vi "WILT Agilent Populate GUI.vi"(7 "Aisle Number":T6=enum."Aisle 1", 8 "Error In":errorcluster, 10 "GUI Aisle Input":T3[](array[typedef]) {"Night Cycle Count" format="%04d"; "Day Cycle Count" format="%04d"}, 11 "Data Array":T1) -> (0 "Error Out":errorcluster, 3 "GUI Aisle Output":T3[](array[typedef]) {"Night Cycle Count" format="%04d"; "Day Cycle Count" format="%04d"}, 5 "Agilent Failure":bool)   [LabVIEW 2016]
uses:
  Type Definitions/WILT Aisle Number.ctl
  Type Definitions/WILT Agilent Channel Definition.ctl
  Type Definitions/WILT DAQ Data.ctl
  Type Definitions/WILT Dryer.ctl
  Type Definitions/WILT Dryer Details.ctl
  Type Definitions/WILT Agilent Data Cluster.ctl
panel:
  out "Index of stations that use\nthe same voltage":string[][](array[string])
  in  "Tab Control":enum32{"Check Information"}(tab)
  out "DAQ Data":T5={"L1 Current"=1.0, "L2 Current"=11.0, "Temperature  Deg F (TC)"=0.0, "Volts"=0.0, "Volts (208)"=0.0, "SW (208)"=0.0}
  out "DAQ Data 2":T5={"L1 Current"=2.0, "L2 Current"=22.0, "Temperature  Deg F (TC)"=0.0, "Volts"=0.0, "Volts (208)"=0.0, "SW (208)"=0.0}
  out "DAQ Data 3":T5={"L1 Current"=3.0, "L2 Current"=33.0, "Temperature  Deg F (TC)"=0.0, "Volts"=0.0, "Volts (208)"=0.0, "SW (208)"=0.0}
  out "DAQ Data 4":T5={"L1 Current"=4.0, "L2 Current"=44.0, "Temperature  Deg F (TC)"=0.0, "Volts"=0.0, "Volts (208)"=0.0, "SW (208)"=0.0}
  out "DAQ Data 5":T5={"L1 Current"=5.0, "L2 Current"=55.0, "Temperature  Deg F (TC)"=0.0, "Volts"=0.0, "Volts (208)"=0.0, "SW (208)"=0.0}
  out "DAQ Data 6":T5={"L1 Current"=6.0, "L2 Current"=66.0, "Temperature  Deg F (TC)"=0.0, "Volts"=0.0, "Volts (208)"=0.0, "SW (208)"=0.0}
  out "DAQ Data 7":T5
  out "DAQ Data 8":T5
  out "DAQ Data 9":T5
  out "DAQ Data 10":T5
  out "DAQ Data 11":T5
  out "DAQ Data 12":T5
  in  "Data Array (Old)":T2[](array[typedef])=[{"Channel"="101", "Station"="1", "Label"="L1 Current", "Agilent Station"="1", "Data"=1.0}, {"Channel"="102", "Station"="1", "Label"="L2 Current", "Agilent Station"="1", "Data"=11.0}, {"Channel"="103", "Station"="2", "Label"="L1 Current", "Agilent Station"="1", "Data"=2.0}, {"Channel"="104", "Station"="2", "Label"="L2 Current", "Agilent Station"="1", "Data"=22.0}, {"Channel"="105", "Station"="3", "Label"="L1 Current", "Agilent Station"="1", "Data"=3.0}, {"Channel"="106", "Station"="3", "Label"="L2 Current", "Agilent Station"="1", "Data"=33.0}, {"Channel"="107", "Station"="4", "Label"="L1 Current", "Agilent Station"="1", "Data"=4.0}, {"Channel"="108", "Station"="4", "Label"="L2 Current", "Agilent Station"="1", "Data"=44.0}, {"Channel"="109", "Station"="5", "Label"="L1 Current", "Agilent Station"="1", "Data"=5.0}, {"Channel"="110", "Station"="5", "Label"="L2 Current", "Agilent Station"="1", "Data"=55.0}, {"Channel"="111", "Station"="6", "Label"="L1 Current", "Agilent Station"="1", "Data"=6.0}, {"Channel"="112", "Station"="6", "Label"="L2 Current", "Agilent Station"="1", "Data"=66.0}, {"Channel"="113", "Station"="7", "Label"="L1 Current", "Agilent Station"="1", "Data"=7.0}, {"Channel"="114", "Station"="7", "Label"="L2 Current", "Agilent Station"="1", "Data"=77.0}, {"Channel"="115", "Station"="8", "Label"="L1 Current", "Agilent Station"="1", "Data"=8.0}, {"Channel"="116", "Station"="8", "Label"="L2 Current", "Agilent Station"="1", "Data"=88.0}, {"Channel"="201", "Station"="9", "Label"="L1 Current", "Agilent Station"="1", "Data"=9.0}, {"Channel"="202", "Station"="9", "Label"="L2 Current", "Agilent Station"="1", "Data"=99.0}, {"Channel"="203", "Station"="10", "Label"="L1 Current", "Agilent Station"="1", "Data"=10.0}, {"Channel"="204", "Station"="10", "Label"="L2 Current", "Agilent Station"="1", "Data"=1010.0}, {"Channel"="205", "Station"="11", "Label"="L1 Current", "Agilent Station"="1", "Data"=11.0}, {"Channel"="206", "Station"="11", "Label"="L2 Current", "Agilent Station"="1", "Data"=1111.0}, {"Channel"="207", "Station"="12", "Label"="L1 Current", "Agilent Station"="1", "Data"=12.0}, {"Channel"="208", "Station"="12", "Label"="L2 Current", "Agilent Station"="1", "Data"=1212.0}, {"Channel"="209", "Station"="13", "Label"="L1 Current", "Agilent Station"="1", "Data"=13.0}, {"Channel"="210", "Station"="13", "Label"="L2 Current", "Agilent Station"="1", "Data"=1313.0}, {"Channel"="211", "Station"="14", "Label"="L1 Current", "Agilent Station"="1", "Data"=14.0}, {"Channel"="212", "Station"="14", "Label"="L2 Current", "Agilent Station"="1", "Data"=1414.0}, {"Channel"="213", "Station"="15", "Label"="L1 Current", "Agilent Station"="1", "Data"=15.0}, {"Channel"="214", "Station"="15", "Label"="L2 Current", "Agilent Station"="1", "Data"=1515.0}, {"Channel"="215", "Station"="16", "Label"="L1 Current", "Agilent Station"="1", "Data"=16.0}, {"Channel"="216", "Station"="16", "Label"="L2 Current", "Agilent Station"="1", "Data"=1616.0}, {"Channel"="301", "Station"="17", "Label"="L1 Current", "Agilent Station"="1", "Data"=17.0}, {"Channel"="302", "Station"="17", "Label"="L2 Current", "Agilent Station"="1", "Data"=1717.0}, {"Channel"="303", "Station"="18", "Label"="L1 Current", "Agilent Station"="1", "Data"=18.0}, {"Channel"="304", "Station"="18", "Label"="L2 Current", "Agilent Station"="1", "Data"=1818.0}, {"Channel"="305", "Station"="19", "Label"="L1 Current", "Agilent Station"="1", "Data"=19.0}, {"Channel"="306", "Station"="19", "Label"="L2 Current", "Agilent Station"="1", "Data"=1919.0}, {"Channel"="307", "Station"="20", "Label"="L1 Current", "Agilent Station"="1", "Data"=0.0}, {"Channel"="308", "Station"="20", "Label"="L2 Current", "Agilent Station"="1", "Data"=0.0}, {"Channel"="309", "Station"="21", "Label"="L1 Current", "Agilent Station"="1", "Data"=0.0}, {"Channel"="310", "Station"="21", "Label"="L2 Current", "Agilent Station"="1", "Data"=0.0}, {"Channel"="311", "Station"="22", "Label"="L1 Current", "Agilent Station"="1", "Data"=0.0}, {"Channel"="312", "Station"="22", "Label"="L2 Current", "Agilent Station"="1", "Data"=0.0}, {"Channel"="313", "Station"="23", "Label"="L1 Current", "Agilent Station"="1", "Data"=0.0}, {"Channel"="314", "Station"="23", "Label"="L2 Current", "Agilent Station"="1", "Data"=0.0}, {"Channel"="315", "Station"="24", "Label"="L1 Current", "Agilent Station"="1", "Data"=0.0}, {"Channel"="316", "Station"="24", "Label"="L2 Current", "Agilent Station"="1", "Data"=0.0}, {"Channel"="101", "Station"="25", "Label"="L1 Current", "Agilent Station"="2", "Data"=0.0}, {"Channel"="102", "Station"="25", "Label"="L2 Current", "Agilent Station"="2", "Data"=0.0}, {"Channel"="103", "Station"="26", "Label"="L1 Current", "Agilent Station"="2", "Data"=0.0}, {"Channel"="104", "Station"="26", "Label"="L2 Current", "Agilent Station"="2", "Data"=0.0}, {"Channel"="105", "Station"="27", "Label"="L1 Current", "Agilent Station"="2", "Data"=0.0}, {"Channel"="106", "Station"="27", "Label"="L2 Current", "Agilent Station"="2", "Data"=0.0}, {"Channel"="107", "Station"="28", "Label"="L1 Current", "Agilent Station"="2", "Data"=0.0}, {"Channel"="108", "Station"="28", "Label"="L2 Current", "Agilent Station"="2", "Data"=0.0}, {"Channel"="109", "Station"="29", "Label"="L1 Current", "Agilent Station"="2", "Data"=0.0}, {"Channel"="110", "Station"="29", "Label"="L2 Current", "Agilent Station"="2", "Data"=0.0}, {"Channel"="111", "Station"="30", "Label"="L1 Current", "Agilent Station"="2", "Data"=0.0}, {"Channel"="112", "Station"="30", "Label"="L2 Current", "Agilent Station"="2", "Data"=0.0}, {"Channel"="113", "Station"="31", "Label"="L1 Current", "Agilent Station"="2", "Data"=0.0}, {"Channel"="114", "Station"="31", "Label"="L2 Current", "Agilent Station"="2", "Data"=0.0}, {"Channel"="115", "Station"="32", "Label"="L1 Current", "Agilent Station"="2", "Data"=0.0}, {"Channel"="116", "Station"="32", "Label"="L2 Current", "Agilent Station"="2", "Data"=0.0}, {"Channel"="201", "Station"="5", "Label"="Volts", "Agilent Station"="2", "Data"=555.0}, {"Channel"="202", "Station"="6", "Label"="Volts", "Agilent Station"="2", "Data"=666.0}, {"Channel"="203", "Station"="7", "Label"="Volts", "Agilent Station"="2", "Data"=777.0}, {"Channel"="204", "Station"="8", "Label"="Volts", "Agilent Station"="2", "Data"=888.0}, {"Channel"="205", "Station"="9", "Label"="Volts", "Agilent Station"="2", "Data"=999.0}, {"Channel"="206", "Station"="10", "Label"="Volts", "Agilent Station"="2", "Data"=101010.0}, {"Channel"="207", "Station"="11", "Label"="Volts", "Agilent Station"="2", "Data"=111111.0}, {"Channel"="208", "Station"="12", "Label"="Volts", "Agilent Station"="2", "Data"=121212.0}, {"Channel"="209", "Station"="13", "Label"="Volts", "Agilent Station"="2", "Data"=0.0}, {"Channel"="210", "Station"="14", "Label"="Volts", "Agilent Station"="2", "Data"=0.0}, {"Channel"="211", "Station"="21-23", "Label"="Volts", "Agilent Station"="2", "Data"=0.0}, {"Channel"="212", "Station"="24-26", "Label"="Volts", "Agilent Station"="2", "Data"=0.0}, {"Channel"="213", "Station"="27-29", "Label"="Volts", "Agilent Station"="2", "Data"=0.0}, {"Channel"="214", "Station"="30-32", "Label"="Volts", "Agilent Station"="2", "Data"=0.0}, {"Channel"="215", "Station"="15", "Label"="Volts", "Agilent Station"="2", "Data"=0.0}, {"Channel"="216", "Station"="16", "Label"="Volts", "Agilent Station"="2", "Data"=0.0}, {"Channel"="201", "Station"="1", "Label"="Temperature", "Agilent Station"="3", "Data"=1.0}, {"Channel"="202", "Station"="2", "Label"="Temperature", "Agilent Station"="3", "Data"=2.0}, {"Channel"="203", "Station"="3", "Label"="Temperature", "Agilent Station"="3", "Data"=3.0}, {"Channel"="204", "Station"="4", "Label"="Temperature", "Agilent Station"="3", "Data"=4.0}, {"Channel"="205", "Station"="5", "Label"="Temperature", "Agilent Station"="3", "Data"=5.0}, {"Channel"="206", "Station"="6", "Label"="Temperature", "Agilent Station"="3", "Data"=6.0}, {"Channel"="207", "Station"="7", "Label"="Temperature", "Agilent Station"="3", "Data"=7.0}, {"Channel"="208", "Station"="8", "Label"="Temperature", "Agilent Station"="3", "Data"=8.0}, {"Channel"="209", "Station"="9", "Label"="Temperature", "Agilent Station"="3", "Data"=9.0}, {"Channel"="210", "Station"="10", "Label"="Temperature", "Agilent Station"="3", "Data"=10.0}, {"Channel"="211", "Station"="11", "Label"="Temperature", "Agilent Station"="3", "Data"=11.0}, {"Channel"="212", "Station"="12", "Label"="Temperature", "Agilent Station"="3", "Data"=12.0}, {"Channel"="213", "Station"="13", "Label"="Temperature", "Agilent Station"="3", "Data"=0.0}, {"Channel"="214", "Station"="14", "Label"="Temperature", "Agilent Station"="3", "Data"=0.0}, {"Channel"="215", "Station"="15", "Label"="Temperature", "Agilent Station"="3", "Data"=0.0}, {"Channel"="216", "Station"="16", "Label"="Temperature", "Agilent Station"="3", "Data"=0.0}, {"Channel"="217", "Station"="17", "Label"="Temperature", "Agilent Station"="3", "Data"=0.0}, {"Channel"="218", "Station"="18", "Label"="Temperature", "Agilent Station"="3", "Data"=0.0}, {"Channel"="219", "Station"="19", "Label"="Temperature", "Agilent Station"="3", "Data"=0.0}, {"Channel"="220", "Station"="20", "Label"="Temperature", "Agilent Station"="3", "Data"=0.0}, {"Channel"="301", "Station"="21", "Label"="Temperature", "Agilent Station"="3", "Data"=0.0}, {"Channel"="302", "Station"="22", "Label"="Temperature", "Agilent Station"="3", "Data"=0.0}, {"Channel"="303", "Station"="23", "Label"="Temperature", "Agilent Station"="3", "Data"=0.0}, {"Channel"="304", "Station"="24", "Label"="Temperature", "Agilent Station"="3", "Data"=0.0}, {"Channel"="305", "Station"="25", "Label"="Temperature", "Agilent Station"="3", "Data"=0.0}, {"Channel"="306", "Station"="26", "Label"="Temperature", "Agilent Station"="3", "Data"=0.0}, {"Channel"="307", "Station"="27", "Label"="Temperature", "Agilent Station"="3", "Data"=0.0}, {"Channel"="308", "Station"="28", "Label"="Temperature", "Agilent Station"="3", "Data"=0.0}, {"Channel"="309", "Station"="29", "Label"="Temperature", "Agilent Station"="3", "Data"=0.0}, {"Channel"="310", "Station"="30", "Label"="Temperature", "Agilent Station"="3", "Data"=0.0}, {"Channel"="311", "Station"="31", "Label"="Temperature", "Agilent Station"="3", "Data"=0.0}, {"Channel"="312", "Station"="32", "Label"="Temperature", "Agilent Station"="3", "Data"=0.0}, {"Channel"="313", "Station"="1", "Label"="Volts", "Agilent Station"="3", "Data"=111.0}, {"Channel"="314", "Station"="2", "Label"="Volts", "Agilent Station"="3", "Data"=222.0}, {"Channel"="315", "Station"="3", "Label"="Volts", "Agilent Station"="3", "Data"=333.0}, {"Channel"="316", "Station"="4", "Label"="Volts", "Agilent Station"="3", "Data"=444.0}, {"Channel"="101", "Station"="33", "Label"="L1 Current", "Agilent Station"="4", "Data"=0.0}, {"Channel"="102", "Station"="33", "Label"="L2 Current", "Agilent Station"="4", "Data"=0.0}, {"Channel"="103", "Station"="34", "Label"="L1 Current", "Agilent Station"="4", "Data"=0.0}, {"Channel"="104", "Station"="34", "Label"="L2 Current", "Agilent Station"="4", "Data"=0.0}, {"Channel"="105", "Station"="35", "Label"="L1 Current", "Agilent Station"="4", "Data"=0.0}, {"Channel"="106", "Station"="35", "Label"="L2 Current", "Agilent Station"="4", "Data"=0.0}, {"Channel"="107", "Station"="36", "Label"="L1 Current", "Agilent Station"="4", "Data"=0.0}, {"Channel"="108", "Station"="36", "Label"="L2 Current", "Agilent Station"="4", "Data"=0.0}, {"Channel"="109", "Station"="37", "Label"="L1 Current", "Agilent Station"="4", "Data"=0.0}, {"Channel"="110", "Station"="37", "Label"="L2 Current", "Agilent Station"="4", "Data"=0.0}, {"Channel"="111", "Station"="38", "Label"="L1 Current", "Agilent Station"="4", "Data"=0.0}, {"Channel"="112", "Station"="38", "Label"="L2 Current", "Agilent Station"="4", "Data"=0.0}, {"Channel"="113", "Station"="39", "Label"="L1 Current", "Agilent Station"="4", "Data"=0.0}, {"Channel"="114", "Station"="39", "Label"="L2 Current", "Agilent Station"="4", "Data"=0.0}, {"Channel"="115", "Station"="40", "Label"="L1 Current", "Agilent Station"="4", "Data"=0.0}, {"Channel"="116", "Station"="40", "Label"="L2 Current", "Agilent Station"="4", "Data"=0.0}, {"Channel"="201", "Station"="41", "Label"="L1 Current", "Agilent Station"="4", "Data"=0.0}, {"Channel"="202", "Station"="41", "Label"="L2 Current", "Agilent Station"="4", "Data"=0.0}, {"Channel"="203", "Station"="42", "Label"="L1 Current", "Agilent Station"="4", "Data"=0.0}, {"Channel"="204", "Station"="42", "Label"="L2 Current", "Agilent Station"="4", "Data"=0.0}, {"Channel"="205", "Station"="43", "Label"="L1 Current", "Agilent Station"="4", "Data"=0.0}, {"Channel"="206", "Station"="43", "Label"="L2 Current", "Agilent Station"="4", "Data"=0.0}, {"Channel"="207", "Station"="44", "Label"="L1 Current", "Agilent Station"="4", "Data"=0.0}, {"Channel"="208", "Station"="44", "Label"="L2 Current", "Agilent Station"="4", "Data"=0.0}, {"Channel"="209", "Station"="45", "Label"="L1 Current", "Agilent Station"="4", "Data"=0.0}, {"Channel"="210", "Station"="45", "Label"="L2 Current", "Agilent Station"="4", "Data"=0.0}, {"Channel"="211", "Station"="46", "Label"="L1 Current", "Agilent Station"="4", "Data"=0.0}, {"Channel"="212", "Station"="46", "Label"="L2 Current", "Agilent Station"="4", "Data"=0.0}, {"Channel"="213", "Station"="47", "Label"="L1 Current", "Agilent Station"="4", "Data"=0.0}, {"Channel"="214", "Station"="47", "Label"="L2 Current", "Agilent Station"="4", "Data"=0.0}, {"Channel"="215", "Station"="48", "Label"="L1 Current", "Agilent Station"="4", "Data"=0.0}, {"Channel"="216", "Station"="48", "Label"="L2 Current", "Agilent Station"="4", "Data"=0.0}, {"Channel"="301", "Station"="49", "Label"="L1 Current", "Agilent Station"="4", "Data"=0.0}, {"Channel"="302", "Station"="49", "Label"="L2 Current", "Agilent Station"="4", "Data"=0.0}, {"Channel"="303", "Station"="50", "Label"="L1 Current", "Agilent Station"="4", "Data"=0.0}, {"Channel"="304", "Station"="50", "Label"="L2 Current", "Agilent Station"="4", "Data"=0.0}, {"Channel"="305", "Station"="51", "Label"="L1 Current", "Agilent Station"="4", "Data"=0.0}, {"Channel"="306", "Station"="51", "Label"="L2 Current", "Agilent Station"="4", "Data"=0.0}, {"Channel"="307", "Station"="52", "Label"="L1 Current", "Agilent Station"="4", "Data"=0.0}, {"Channel"="308", "Station"="52", "Label"="L2 Current", "Agilent Station"="4", "Data"=0.0}, {"Channel"="309", "Station"="53", "Label"="L1 Current", "Agilent Station"="4", "Data"=0.0}, {"Channel"="310", "Station"="53", "Label"="L2 Current", "Agilent Station"="4", "Data"=0.0}, {"Channel"="311", "Station"="54", "Label"="L1 Current", "Agilent Station"="4", "Data"=0.0}, {"Channel"="312", "Station"="54", "Label"="L2 Current", "Agilent Station"="4", "Data"=0.0}, {"Channel"="313", "Station"="55", "Label"="L1 Current", "Agilent Station"="4", "Data"=0.0}, {"Channel"="314", "Station"="55", "Label"="L2 Current", "Agilent Station"="4", "Data"=0.0}, {"Channel"="315", "Station"="56", "Label"="L1 Current", "Agilent Station"="4", "Data"=0.0}, {"Channel"="316", "Station"="56", "Label"="L2 Current", "Agilent Station"="4", "Data"=0.0}, {"Channel"="101", "Station"="33", "Label"="Temperature", "Agilent Station"="6", "Data"=0.0}, {"Channel"="102", "Station"="34", "Label"="Temperature", "Agilent Station"="6", "Data"=0.0}, {"Channel"="103", "Station"="35", "Label"="Temperature", "Agilent Station"="6", "Data"=0.0}, {"Channel"="104", "Station"="36", "Label"="Temperature", "Agilent Station"="6", "Data"=0.0}, {"Channel"="105", "Station"="37", "Label"="Temperature", "Agilent Station"="6", "Data"=0.0}, {"Channel"="106", "Station"="38", "Label"="Temperature", "Agilent Station"="6", "Data"=0.0}, {"Channel"="107", "Station"="39", "Label"="Temperature", "Agilent Station"="6", "Data"=0.0}, {"Channel"="108", "Station"="40", "Label"="Temperature", "Agilent Station"="6", "Data"=0.0}, {"Channel"="109", "Station"="41", "Label"="Temperature", "Agilent Station"="6", "Data"=0.0}, {"Channel"="110", "Station"="42", "Label"="Temperature", "Agilent Station"="6", "Data"=0.0}, {"Channel"="111", "Station"="43", "Label"="Temperature", "Agilent Station"="6", "Data"=0.0}, {"Channel"="112", "Station"="44", "Label"="Temperature", "Agilent Station"="6", "Data"=0.0}, {"Channel"="113", "Station"="45", "Label"="Temperature", "Agilent Station"="6", "Data"=0.0}, {"Channel"="114", "Station"="46", "Label"="Temperature", "Agilent Station"="6", "Data"=0.0}, {"Channel"="115", "Station"="47", "Label"="Temperature", "Agilent Station"="6", "Data"=0.0}, {"Channel"="116", "Station"="48", "Label"="Temperature", "Agilent Station"="6", "Data"=0.0}, {"Channel"="117", "Station"="49", "Label"="Temperature", "Agilent Station"="6", "Data"=0.0}, {"Channel"="118", "Station"="50", "Label"="Temperature", "Agilent Station"="6", "Data"=0.0}, {"Channel"="119", "Station"="51", "Label"="Temperature", "Agilent Station"="6", "Data"=0.0}, {"Channel"="120", "Station"="52", "Label"="Temperature", "Agilent Station"="6", "Data"=0.0}, {"Channel"="201", "Station"="53", "Label"="Temperature", "Agilent Station"="6", "Data"=0.0}, {"Channel"="202", "Station"="54", "Label"="Temperature", "Agilent Station"="6", "Data"=0.0}, {"Channel"="203", "Station"="55", "Label"="Temperature", "Agilent Station"="6", "Data"=0.0}, {"Channel"="204", "Station"="56", "Label"="Temperature", "Agilent Station"="6", "Data"=0.0}, {"Channel"="205", "Station"="33-35", "Label"="Volts", "Agilent Station"="6", "Data"=0.0}, {"Channel"="206", "Station"="36-38", "Label"="Volts", "Agilent Station"="6", "Data"=0.0}, {"Channel"="207", "Station"="39-40", "Label"="Volts", "Agilent Station"="6", "Data"=0.0}, {"Channel"="208", "Station"="42-44", "Label"="Volts", "Agilent Station"="6", "Data"=0.0}, {"Channel"="209", "Station"="45-47", "Label"="Volts", "Agilent Station"="6", "Data"=0.0}, {"Channel"="210", "Station"="45", "Label"="Volts (208)", "Agilent Station"="6", "Data"=0.0}, {"Channel"="211", "Station"="45", "Label"="SW (208)", "Agilent Station"="6", "Data"=0.0}, {"Channel"="212", "Station"="48-50", "Label"="Volts", "Agilent Station"="6", "Data"=0.0}, {"Channel"="213", "Station"="48", "Label"="SW (208)", "Agilent Station"="6", "Data"=0.0}, {"Channel"="214", "Station"="51", "Label"="Volts (208)", "Agilent Station"="6", "Data"=0.0}, {"Channel"="215", "Station"="51", "Label"="SW (208)", "Agilent Station"="6", "Data"=0.0}, {"Channel"="216", "Station"="54-56", "Label"="Volts", "Agilent Station"="6", "Data"=0.0}, {"Channel"="301", "Station"="17", "Label"="Volts", "Agilent Station"="6", "Data"=0.0}, {"Channel"="302", "Station"="18", "Label"="Volts", "Agilent Station"="6", "Data"=0.0}, {"Channel"="303", "Station"="19", "Label"="Volts", "Agilent Station"="6", "Data"=0.0}, {"Channel"="304", "Station"="20", "Label"="Volts", "Agilent Station"="6", "Data"=0.0}, {"Channel"="305", "Station"="51-53", "Label"="Volts", "Agilent Station"="6", "Data"=0.0}, {"Channel"="306", "Station"="48", "Label"="Volts (208)", "Agilent Station"="6", "Data"=0.0}]
  # "Day"
  # "Night"
  # "Day"
  # "Night"
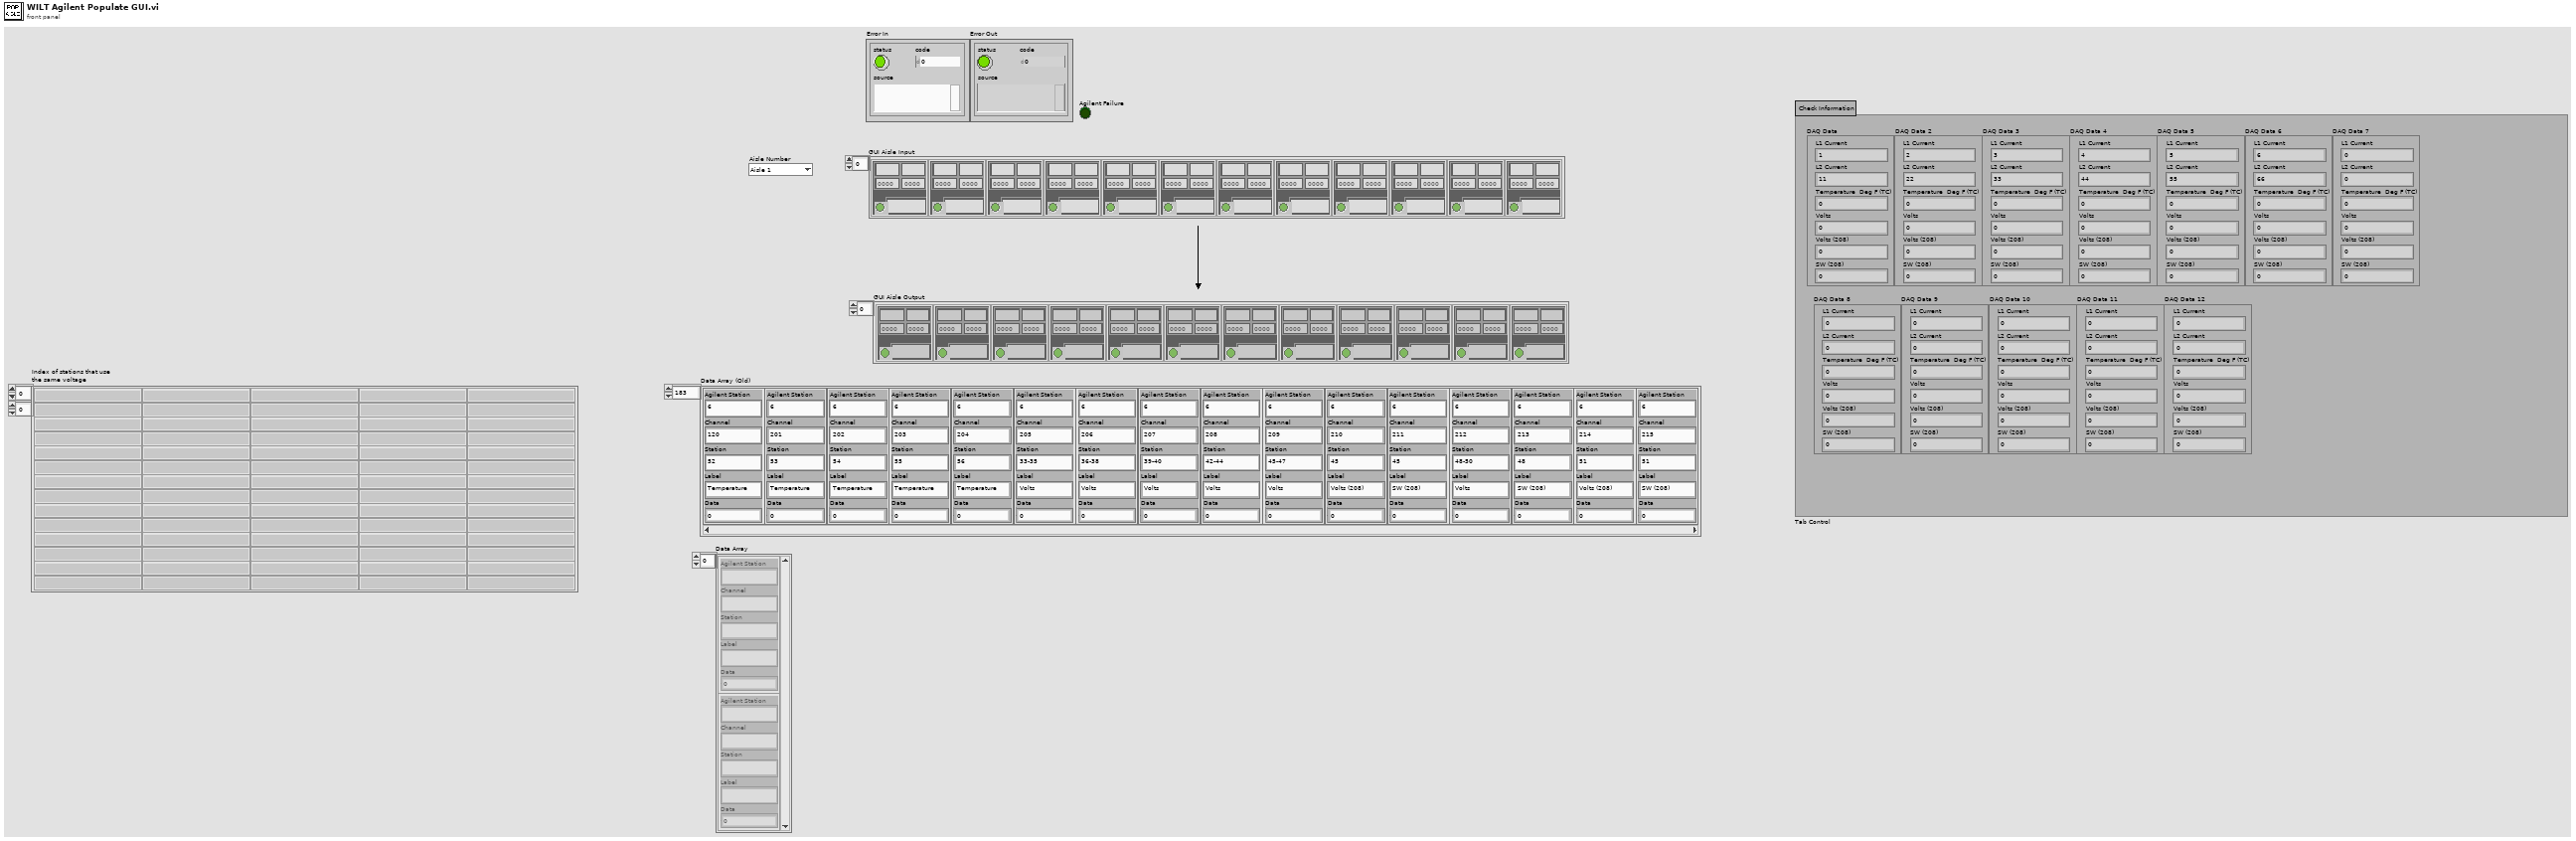
[diagram p1: front panel]
types:
  T1 = typedef "WILT Agilent Data Cluster.ctl" = T2[]
  T2 = typedef "WILT Agilent Channel Definition.ctl" = cluster{"Channel":string, "Station":string, "Label":string, "Agilent Station":string, "Data":dbl}
  T3 = typedef "WILT Dryer.ctl" = cluster{"Lab ID":string, "Day Cycle Count":i32, "Station Label":string, "Dryer Details":T4, "Status Color":u32, "Invisible Button":bool, "Night Cycle Count":i32, "Station Index":i32, "Cycle Index":string, "Audit Alert":bool, "Agilent Channel Definition":T2, "DAQ Data":T5}
  T4 = typedef "WILT Dryer Details.ctl" = cluster{"Station":string, "Lab ID":string, "TR Number":string}
  T5 = typedef "WILT DAQ Data.ctl" = cluster{"L1 Current":dbl, "L2 Current":dbl, "Temperature  Deg F (TC)":dbl, "Volts":dbl, "Volts (208)":dbl, "SW (208)":dbl}
  T6 = typedef "WILT Aisle Number.ctl" = enum16{"Aisle 4", "Aisle 3", "Aisle 2", "Aisle 1A", "Aisle 1"}
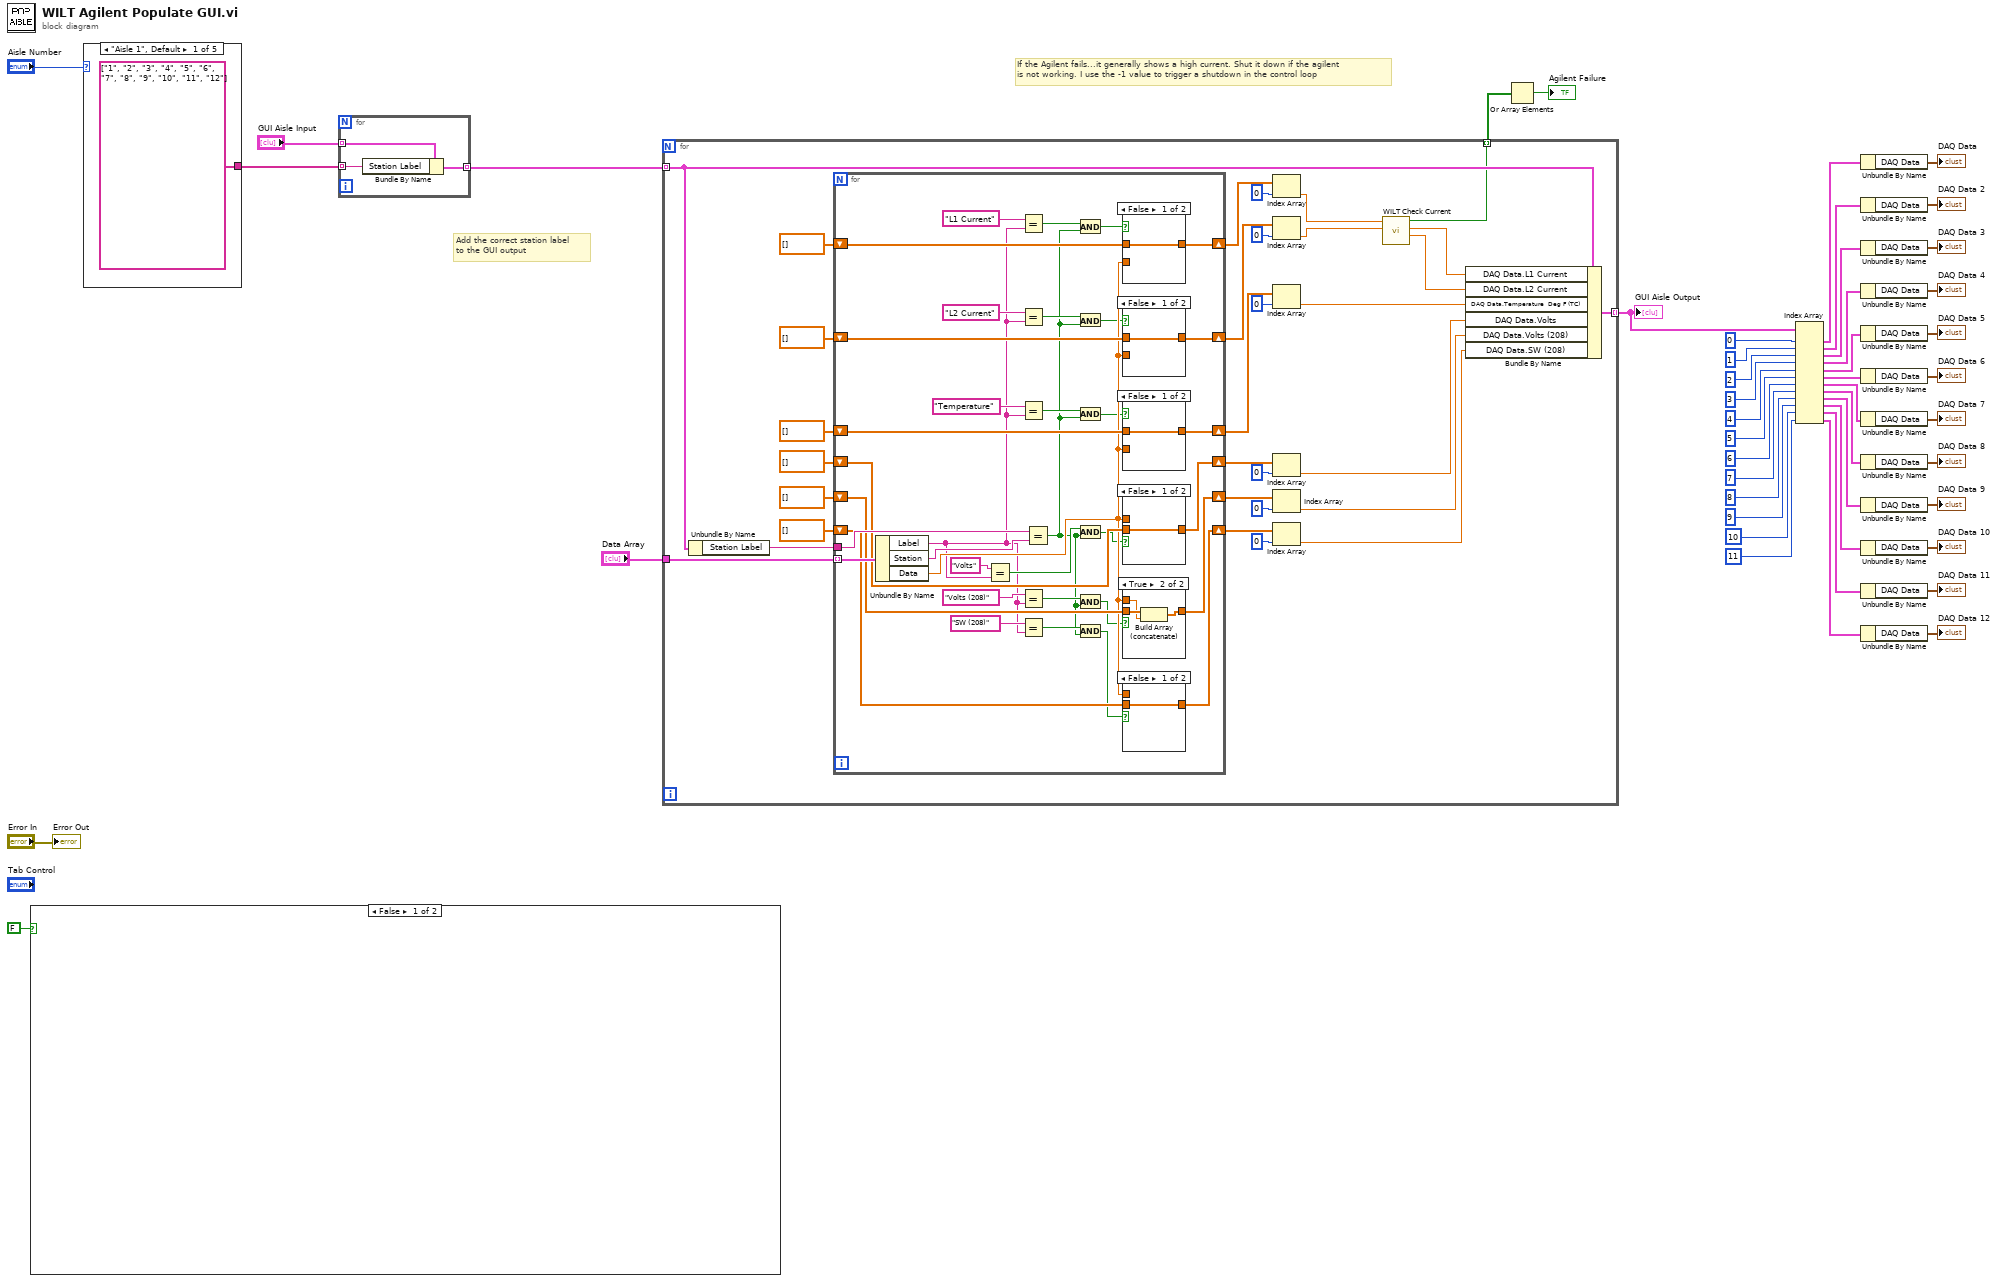
[diagram p0: block diagram]
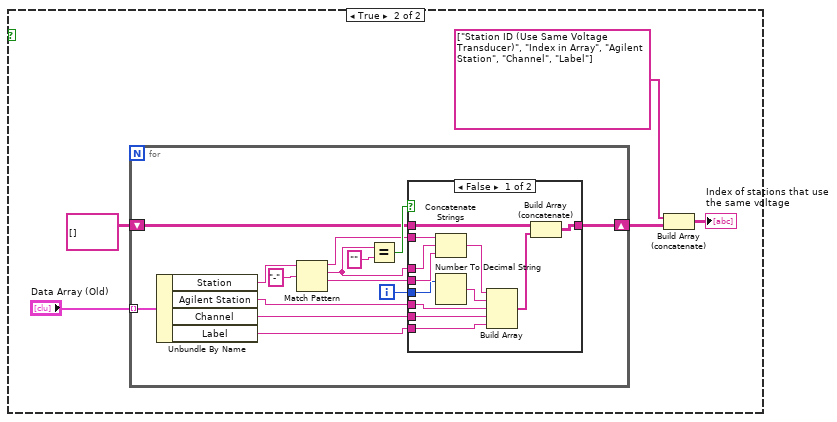
[diagram p2: hidden frame]
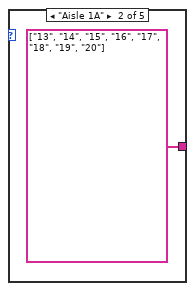
[diagram p4: hidden frame]
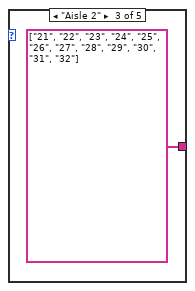
[diagram p5: hidden frame]
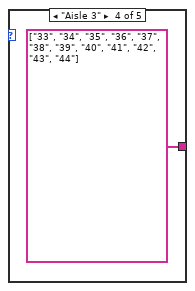
[diagram p6: hidden frame]
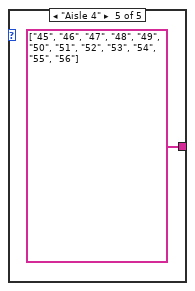
[diagram p7: hidden frame]
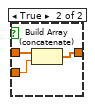
[diagram p8: hidden frame]
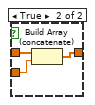
[diagram p9: hidden frame]
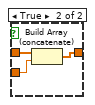
[diagram p10: hidden frame]
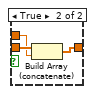
[diagram p11: hidden frame]
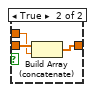
[diagram p13: hidden frame]
diagram:
  # "If the Agilent fails...it generally shows a high current. Shut it down if the agilent \nis not working. I use the -1 value to trigger a shutdown in the control loop"
  # "Add the correct station label\nto the GUI output"
  n1 = case shown="False" FALSE {
    frame False {
    }
    frame True {
      n2 = for {
        tunnel: "Data Array (Old)" -> [w65] mode=indexing
        shift-right: [w55] -> w48
        shift-left: string[][] [] -> [w60]
        i -> [w56]
        n3 = Unbundle By Name(w65) -> ("Station"=w64:string, "Agilent Station"=w54:string, "Channel"=w53:string, "Label"=w52:string)
        n4 = Match Pattern(string=w64, regular expression="-") -> (before substring=w58:string, match substring=w59:string, after substring=w57:string)  [unwired: 1 in, 1 out]
        n5 = Equal?(x=w59, y="") -> (x = y?=w62:bool)
        n6 = case shown="False" w62 {
          tunnel: w60 -> [w77 w78]
          tunnel: [w72 w78] -> w55
          tunnel: w59 -> [w75 _]
          tunnel: w58 -> [w76 _]
          tunnel: w57 -> [w74 _]
          tunnel: w56 -> [w73 _]
          tunnel: w54 -> [w68 _]
          tunnel: w53 -> [w67 _]
          tunnel: w52 -> [w66 _]
          frame False {
            n7 = Concatenate Strings(w76, w75, w74) -> (w71:string)
            n8 = Number To Decimal String(number=w73) -> (decimal integer string=w70:string)  [unwired: 1 in]
            n9 = Build Array(w71, w70, w68, w67, w66) -> (w69:string[])
            n10 = Build Array (concatenate)(w77, w69) -> (w72:string[][])
          }
          frame True {
          }
        }
      }
      n11 = Build Array (concatenate)(string[] ["Station ID (Use Same Voltage Transducer)", "Index in Array", "Agilent Station", "Channel", "Label"], w48) -> (→"Index of stations that use\nthe same voltage":string[][])
    }
  }
  n12 = case shown="\"Aisle 1\", Default" "Aisle Number" {
    tunnel: [string[] ["1", "2", "3", "4", "5", "6", "7", "8", "9", "10", "11", "12"] string[] ["13", "14", "15", "16", "17", "18", "19", "20"] string[] ["21", "22", "23", "24", "25", "26", "27", "28", "29", "30", "31", "32"] string[] ["33", "34", "35", "36", "37", "38", "39", "40", "41", "42", "43", "44"] string[] ["45", "46", "47", "48", "49", "50", "51", "52", "53", "54", "55", "56"]] -> w45
    frame "Aisle 1", Default {
    }
    frame "Aisle 1A" {
    }
    frame "Aisle 2" {
    }
    frame "Aisle 3" {
    }
    frame "Aisle 4" {
    }
  }
  n13 = for {
    tunnel: "GUI Aisle Input" -> [w86] mode=indexing
    tunnel: w45 -> [w85] mode=indexing
    tunnel: [w84] -> w44 mode=indexing
    n14 = Bundle By Name(cluster=w86, "Station Label"=w85) -> (w84:T3)
  }
  n15 = for {
    tunnel: w44 -> [w115] mode=indexing
    tunnel: [w117] -> w43 mode=indexing
    tunnel: "Data Array" -> [w113]
    tunnel: [w87] -> w2 mode=indexing
    n16 = Unbundle By Name(w115) -> ("Station Label"=w114:string)
    n17 = for {
      tunnel: w113 -> [w153] mode=indexing
      tunnel: w114 -> [w151]
      shift-right: [w149] -> w107
      shift-left: dbl[] [] -> [w150]
      shift-right: [w147] -> w104
      shift-left: dbl[] [] -> [w148]
      shift-right: [w145] -> w101
      shift-left: dbl[] [] -> [w146]
      shift-right: [w143] -> w98
      shift-left: dbl[] [] -> [w144]
      shift-right: [w141] -> w95
      shift-left: dbl[] [] -> [w142]
      shift-right: [w138] -> w93
      shift-left: dbl[] [] -> [w140]
      n18 = Unbundle By Name(w153) -> ("Label"=w119:string, "Station"=w152:string, "Data"=w139:dbl)
      n19 = Equal?(x="Volts", y=w119) -> (x = y?=w132:bool)
      n20 = Equal?(x="L1 Current", y=w119) -> (x = y?=w126:bool)
      n21 = Equal?(x="L2 Current", y=w119) -> (x = y?=w128:bool)
      n22 = Equal?(x="Temperature", y=w119) -> (x = y?=w130:bool)
      n23 = Equal?(x="Volts (208)", y=w119) -> (x = y?=w134:bool)
      n24 = Equal?(x="SW (208)", y=w119) -> (x = y?=w136:bool)
      n25 = Equal?(x=w151, y=w152) -> (x = y?=w118:bool)
      n26 = And(x=w126, y=w118) -> (x .and. y?=w125:bool)
      n27 = And(x=w128, y=w118) -> (x .and. y?=w127:bool)
      n28 = And(x=w130, y=w118) -> (x .and. y?=w129:bool)
      n29 = And(x=w132, y=w118) -> (x .and. y?=w131:bool)
      n30 = And(x=w134, y=w118) -> (x .and. y?=w133:bool)
      n31 = And(x=w136, y=w118) -> (x .and. y?=w137:bool)
      n32 = case shown="False" w125 {
        tunnel: w140 -> [w154 w157]
        tunnel: [w154 w156] -> w138
        tunnel: w139 -> [_ w155]
        frame False {
        }
        frame True {
          n33 = Build Array (concatenate)(w157, w155) -> (w156:dbl[])
        }
      }
      n34 = case shown="False" w127 {
        tunnel: w142 -> [w158 w161]
        tunnel: [w158 w160] -> w141
        tunnel: w139 -> [_ w159]
        frame False {
        }
        frame True {
          n35 = Build Array (concatenate)(w161, w159) -> (w160:dbl[])
        }
      }
      n36 = case shown="False" w129 {
        tunnel: w144 -> [w162 w165]
        tunnel: [w162 w164] -> w143
        tunnel: w139 -> [_ w163]
        frame False {
        }
        frame True {
          n37 = Build Array (concatenate)(w165, w163) -> (w164:dbl[])
        }
      }
      n38 = case shown="False" w131 {
        tunnel: w146 -> [w166 w169]
        tunnel: [w166 w168] -> w145
        tunnel: w139 -> [_ w167]
        frame False {
        }
        frame True {
          n39 = Build Array (concatenate)(w169, w167) -> (w168:dbl[])
        }
      }
      n40 = case shown="True" w133 {
        tunnel: w148 -> [w170 w173]
        tunnel: [w170 w172] -> w147
        tunnel: w139 -> [_ w171]
        frame False {
        }
        frame True {
          n41 = Build Array (concatenate)(w173, w171) -> (w172:dbl[])
        }
      }
      n42 = case shown="False" w137 {
        tunnel: w150 -> [w174 w177]
        tunnel: [w174 w176] -> w149
        tunnel: w139 -> [_ w175]
        frame False {
        }
        frame True {
          n43 = Build Array (concatenate)(w177, w175) -> (w176:dbl[])
        }
      }
    }
    n44 = Index Array(array=w93, index=0) -> (element=w91:dbl)
    n45 = Index Array(array=w95, index=0) -> (element=w89:dbl)
    n46 = Index Array(array=w98, index=0) -> (element=w96:dbl)
    n47 = Index Array(array=w101, index=0) -> (element=w99:dbl)
    n48 = Index Array(array=w104, index=0) -> (element=w102:dbl)
    n49 = Index Array(array=w107, index=0) -> (element=w105:dbl)
    n50 = call "WILT Check Current.vi"("L2 Current"=w89, "L1 Current"=w91) -> ("L2 Current Out"=w88:dbl, "L1 Current Out"=w90:dbl, "Agilent Failure"=w87:bool)  [unwired: 7 in]
    n51 = Bundle By Name(cluster=w115, "DAQ Data.L1 Current"=w90, "DAQ Data.L2 Current"=w88, "DAQ Data.Temperature  Deg F (TC)"=w96, "DAQ Data.Volts"=w99, "DAQ Data.Volts (208)"=w102, "DAQ Data.SW (208)"=w105) -> (w117:T3)
  }
  "GUI Aisle Output" <- w43
  n52 = Or Array Elements(Boolean array=w2) -> (logical OR=→"Agilent Failure":bool)
  n53 = Index Array(array=w43, index #1=0 ("index"), index #2=1 ("index"), index #3=2 ("index"), index #4=3 ("index"), index #5=4 ("index"), index #6=5 ("index"), index #7=6 ("index"), index #8=7 ("index"), index #9=8 ("index"), index #10=9 ("index"), index #11=10 ("index"), index #12=11 ("index")) -> (element #1=w42:T3, element #2=w38:T3, element #3=w26:T3, element #4=w25:T3, element #5=w24:T3, element #6=w23:T3, element #7=w22:T3, element #8=w21:T3, element #9=w20:T3, element #10=w19:T3, element #11=w18:T3, element #12=w17:T3)
  n54 = Unbundle By Name(w42) -> ("DAQ Data"=→"DAQ Data":T5)
  n55 = Unbundle By Name(w38) -> ("DAQ Data"=→"DAQ Data 2":T5)
  n56 = Unbundle By Name(w26) -> ("DAQ Data"=→"DAQ Data 3":T5)
  n57 = Unbundle By Name(w25) -> ("DAQ Data"=→"DAQ Data 4":T5)
  n58 = Unbundle By Name(w24) -> ("DAQ Data"=→"DAQ Data 5":T5)
  n59 = Unbundle By Name(w23) -> ("DAQ Data"=→"DAQ Data 6":T5)
  n60 = Unbundle By Name(w22) -> ("DAQ Data"=→"DAQ Data 7":T5)
  n61 = Unbundle By Name(w21) -> ("DAQ Data"=→"DAQ Data 8":T5)
  n62 = Unbundle By Name(w20) -> ("DAQ Data"=→"DAQ Data 9":T5)
  n63 = Unbundle By Name(w19) -> ("DAQ Data"=→"DAQ Data 10":T5)
  n64 = Unbundle By Name(w18) -> ("DAQ Data"=→"DAQ Data 11":T5)
  n65 = Unbundle By Name(w17) -> ("DAQ Data"=→"DAQ Data 12":T5)
  "Error Out" <- "Error In"
